vi "cruise control.vi"(9 "Cruise type":enum16{"Off", "On cruise", "On limit"}(ring), 10 "speed limit":i16, 11 "Array":T1[](array[typedef]) {"Data" format="%.0x"}) -> (3 "Array 2":T1[](array[typedef]) {"Data" format="%.0x"})   [LabVIEW 2021, in "uCanDriver.lvlib" / "uCAN.lvclass"]
uses:
  uCAN.lvclass
  typedefs/frame.ctl
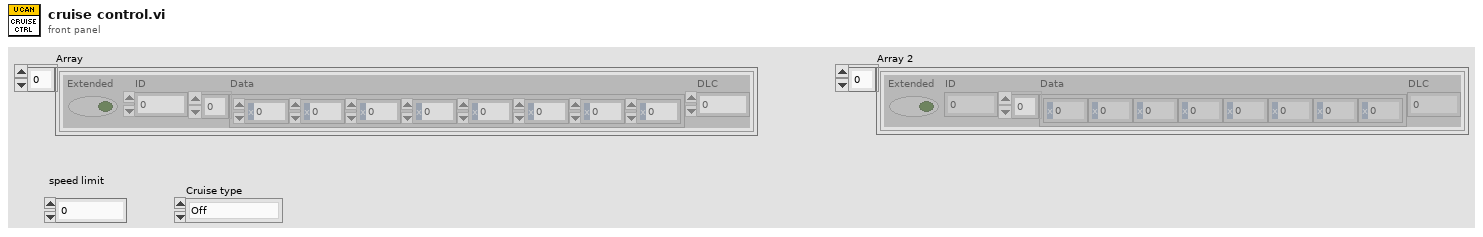
[diagram p1: front panel]
types:
  T1 = typedef "uCanDriver.lvlib/uCAN.lvclass/frame.ctl" = cluster{"Extended":bool, "ID":u32, "Data":u8[], "DLC":u8}
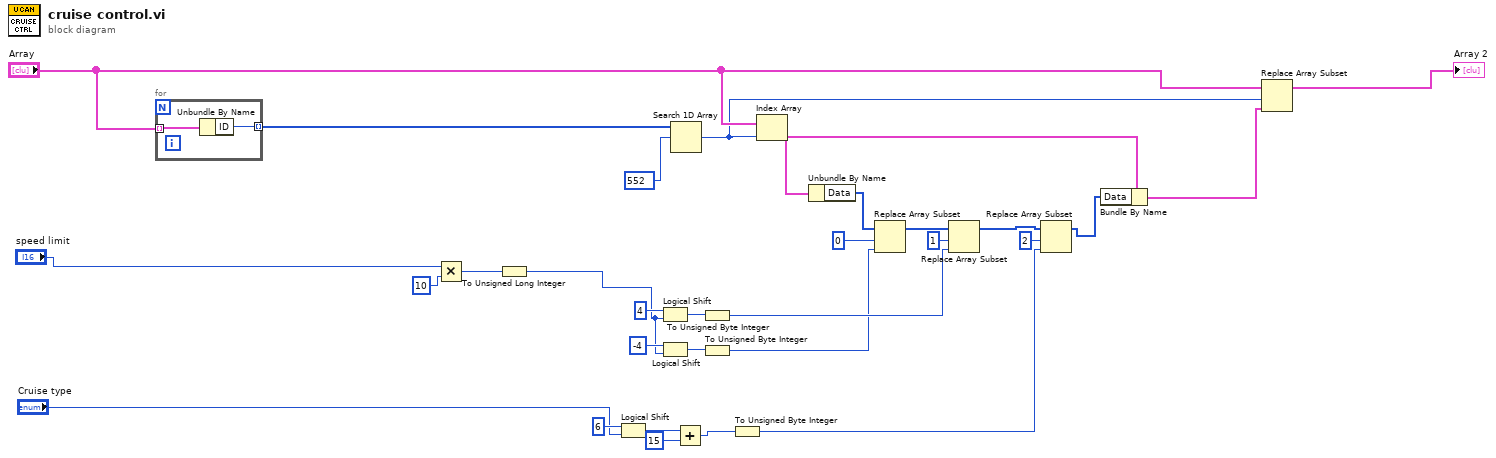
[diagram p0: block diagram]
diagram:
  n1 = for {
    tunnel: "Array" -> [w32] mode=indexing
    tunnel: [w31] -> w28 mode=indexing
    n2 = Unbundle By Name(w32) -> ("ID"=w31:u32)
  }
  n3 = Multiply(x="speed limit", y=i16 10) -> (x*y=w8:i16)
  n4 = To Unsigned Long Integer(number=w8) -> (unsigned 32bit integer=w7:u32)
  n5 = Logical Shift(y=i16 6, x="Cruise type") -> (x << y=w6:u32)
  n6 = Logical Shift(y=i16 4, x=w7) -> (x << y=w18:u32)
  n7 = Logical Shift(y=i16 -4, x=w7) -> (x << y=w12:u32)
  n8 = Search 1D Array(1D array=w28, element=u32 552) -> (index of element=w26:i32)  [unwired: 1 in]
  n9 = Add(x=w6, y=u32 15) -> (x+y=w3:u32)
  n10 = To Unsigned Byte Integer(number=w18) -> (unsigned 8bit integer=w10:u8)
  n11 = To Unsigned Byte Integer(number=w12) -> (unsigned 8bit integer=w9:u8)
  n12 = To Unsigned Byte Integer(number=w3) -> (unsigned 8bit integer=w1:u8)
  n13 = Index Array(array="Array", index=w26) -> (element=w30:T1)
  n14 = Unbundle By Name(w30) -> ("Data"=w22:u8[])
  n15 = Replace Array Subset(array=w22, new element=w9, index=0) -> (w21:u8[])
  n16 = Replace Array Subset(array=w21, new element=w10, index=1) -> (w13:u8[])
  n17 = Replace Array Subset(array=w13, new element=w1, index=2) -> (w14:u8[])
  n18 = Bundle By Name(cluster=w30, "Data"=w14) -> (w24:T1)
  n19 = Replace Array Subset(array="Array", new element=w24, index=w26) -> (→"Array 2":T1[])
